vi "ExampleServer.vi"() -> ()   [LabVIEW 2013, in "Tag Bus Web Interface tests.lvlib"]
uses:
  Tag Bus Web Interface tests.lvlib
  execution/Tag Bus Web Interface runtime.lvclass
  configuration/Tag Bus Web Interface configuration.lvclass
  <vilib>/NI/Tag Bus/tag/Data Type.ctl
  <vilib>/NI/Tag Bus Module Framework/channel/channel classification.ctl
  <vilib>/NI/Tag Bus/table/data polymorphs/write one/write Double.vi
  <vilib>/NI/Tag Bus/table/data polymorphs/read one/read Boolean.vi
  <vilib>/NI/Tag Bus/table/data table.lvlib
  <vilib>/NI/Tag Bus Module Framework/channel/TBM channel.lvclass
  <vilib>/NI/Tag Bus/tag/tag descriptor.lvclass
panel:
  out "Bool0":bool
  in  "Dbl0":dbl
  in  "stop":bool
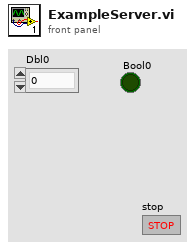
[diagram p1: front panel]
types:
  T1 = typedef "TBM channel.lvclass/channel classification.ctl" = enum16{"input data", "output data", "processing parameter", "processing result"}
  T2 = typedef "tag bus.lvlib/tag descriptor.lvclass/Data Type.ctl" = enum16{"Double", "Single", "I64", "I32", "I16", "I8", "U64", "U32", "U16", "U8", "Boolean", "String", "Array of Double", "Array of Single", "Array of I64", "Array of I32", "Array of I16", "Array of I8", "Array of U64", "Array of U32", "Array of U16", "Array of U8", "Array of Boolean", "Array of String"}
  T3 = typedef "TBM channel.lvclass/data tables.ctl" = cluster{"input data":T4, "processing parameter":T4, "processing result":T4, "output data":T4}
  T4 = typedef "tag bus.lvlib/dictionary table pair.ctl" = cluster{"data dictionary":refnum<class "data dictionary.lvclass">, "data table":T5}
  T5 = typedef "tag bus.lvlib/data table.lvlib/data table.ctl" = cluster{"Double":dbl[], "Single":sgl[], "I64":i64[], "I32":i32[], "I16":i16[], "I8":i8[], "U64":u64[], "U32":u32[], "U16":u16[], "U8":u8[], "Boolean":bool[], "String":string[], "Array of Double":cluster{"DBL Array":dbl[]}[], "Array of Single":cluster{"SGL Array":sgl[]}[], "Array of I64":cluster{"I64 Array":i64[]}[], "Array of I32":cluster{"I32 Array":i32[]}[], "Array of I16":cluster{"I16 Array":i16[]}[], "Array of I8":cluster{"I8 Array":i8[]}[], "Array of U64":cluster{"U64 Array":u64[]}[], "Array of U32":cluster{"U32 Array":u32[]}[], "Array of U16":cluster{"U16 Array":u16[]}[], "Array of U8":cluster{"U8 Array":u8[]}[], "Array of Boolean":cluster{"Boolean Array":bool[]}[], "Array of String":cluster{"String Array":string[]}[]}
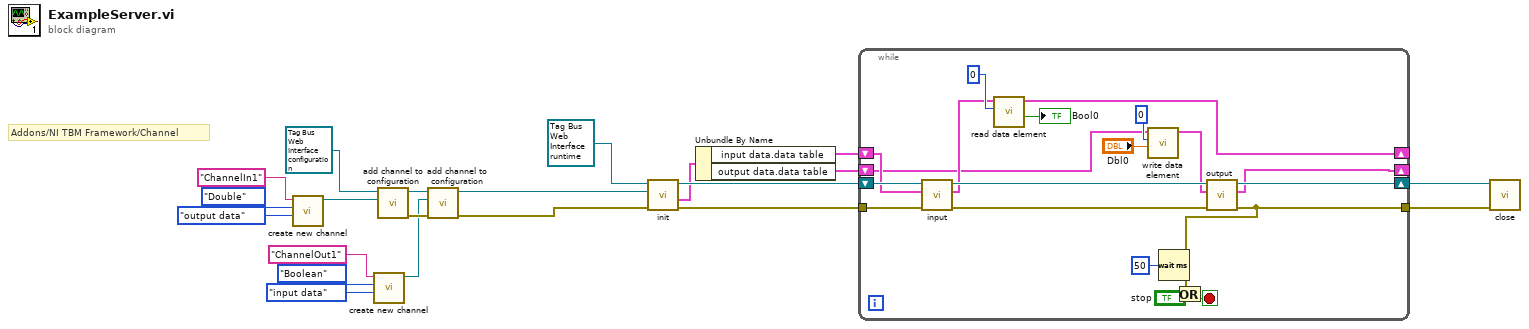
[diagram p0: block diagram]
diagram:
  # "Addons/NI TBM Framework/Channel"
  n1 = call <vilib>:"create new channel.vi"("channel classification"=channel_classification."output data", "data type"=Data_Type."Double", "channel name"="ChannelIn1") -> ("channel"=w4:refnum<class "TBM channel.lvclass">)  [unwired: 8 in]
  n2 = call <vilib>:"create new channel.vi"("channel classification"=channel_classification."input data", "data type"=Data_Type."Boolean", "channel name"="ChannelOut1") -> ("channel"=w3:refnum<class "TBM channel.lvclass">)  [unwired: 8 in]
  n3 = call "add channel to configuration.vi"("TBM channel in"=w4, "Tag Bus Web Interface configuration in"=refnum<class "Tag Bus Web Interface configuration.lvclass"> refnum ("Tag Bus Web Interface configuration")) -> ("error out"=w7:errorcluster, "Tag Bus Web Interface configuration out"=w6:refnum<class "Tag Bus Web Interface configuration.lvclass">)  [unwired: 8 in]
  n4 = call "add channel to configuration.vi"("error in"=w7, "TBM channel in"=w3, "Tag Bus Web Interface configuration in"=w6) -> ("error out"=w1:errorcluster, "Tag Bus Web Interface configuration out"=w2:refnum<class "Tag Bus Web Interface configuration.lvclass">)  [unwired: 7 in]
  n5 = call-dynamic "init.vi"("error in"=w1, "TBM module configuration in"=w2, "Tag Bus Web Interface runtime in"=refnum<class "Tag Bus Web Interface runtime.lvclass"> refnum ("Tag Bus Web Interface runtime")) -> ("error out"=w19:errorcluster, "data allocations"=w14:T3, "Tag Bus Web Interface runtime out"=w20:refnum<class "Tag Bus Web Interface runtime.lvclass">)  [unwired: 5 in, 1 out]
  n6 = Unbundle By Name(w14) -> ("input data.data table"=w16:T5, "output data.data table"=w15:T5)
  n7 = while {
    tunnel: w19 -> [w39]
    tunnel: [w22] -> w17
    shift-right: [w29] -> _
    shift-left: w16 -> [w32]
    shift-right: [w24] -> _
    shift-left: w15 -> [w26]
    shift-right: [w36] -> w18
    shift-left: w20 -> [w40]
    stop <- w23 stop-if-true
    n8 = call-dynamic "input.vi"("error in"=w39, "data table in"=w32, "Tag Bus Web Interface runtime in"=w40) -> ("error out"=w37:errorcluster, "data table out"=w30:T5, "Tag Bus Web Interface runtime out"=w38:refnum<class "Tag Bus Web Interface runtime.lvclass">)  [unwired: 6 in]
    n9 = call-poly <vilib>:"read data element.vi"("index"=0, "data table in"=w30) -> ("value"=→"Bool0":bool, "data table out"=w29:T5)  [unwired: 8 in]
    n10 = call-poly <vilib>:"write data element.vi"("value"="Dbl0", "index"=0, "data table in"=w26) -> ("data table out"=w25:T5)  [unwired: 8 in]
    n11 = Wait (ms)(milliseconds to wait=u32 50) -> ()  [unwired: 1 out]
    n12 = call-dynamic "output.vi"("error in"=w37, "data table in"=w25, "Tag Bus Web Interface runtime in"=w38) -> ("error out"=w22:errorcluster, "data table out"=w24:T5, "Tag Bus Web Interface runtime out"=w36:refnum<class "Tag Bus Web Interface runtime.lvclass">)  [unwired: 6 in]
    n13 = Or(x=w22, y="stop") -> (x .or. y?=w23:bool)
  }
  n14 = call-dynamic "close.vi"("error in"=w17, "Tag Bus Web Interface runtime in"=w18) -> ()  [unwired: 9 in, 1 out]
